vi "Read Port.vi"(8 "error in (no error)":errorcluster, 11 "TCP slave in":refnum<class "TCP Slave.lvclass">) -> (0 "error out":errorcluster, 2 "port":u16, 3 "TCP slave out":refnum<class "TCP Slave.lvclass">)   [LabVIEW 2017, in "SubVIs.lvlib" / "TCP Slave.lvclass"]
doc: "Property accessor for the TCP port."
uses:
  <vilib>/Modbus/subvis/Protocol/TCP/TCP Slave/TCP Slave.lvclass
  <vilib>/Modbus/subvis/Protocol/TCP/TCP Slave/TCP Slave.lvclass/TCP Slave.ctl
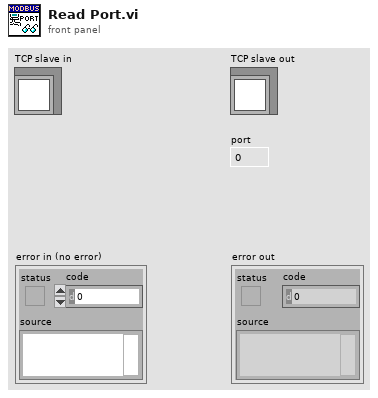
[diagram p1: front panel]
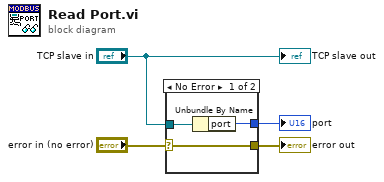
[diagram p0: block diagram]
diagram:
  n1 = case shown="No Error" "error in (no error)" {
    selector: "error in (no error)" -> [w5 w8]
    tunnel: "TCP slave in" -> [w7 _]
    tunnel: [w6 _] -> w3
    tunnel: [w5 w8] -> w1
    frame No Error {
      n2 = Unbundle By Name(w7) -> ("port"=w6:u16)
    }
    frame Error {
    }
  }
  "error out" <- w1
  "port" <- w3
  "TCP slave out" <- "TCP slave in"
